vi "Get board layout.vi"(11 "Board in":refnum<class "Board.lvclass">) -> (2 "Board layout":cluster{"Occupied":bool, "Piece":T1}[][](array[cluster]), 3 "Board out":refnum<class "Board.lvclass">)   [LabVIEW 2015, in "Chesslib.lvlib" / "Board.lvclass"]
uses:
  Board.lvclass
  typedef/Piece.ctl
  typedef/Color.ctl
  typedef/Piece type.ctl
  Pieces/Piece/Piece.lvclass/Piece.ctl
  Pieces/Piece/Piece.lvclass
  Chesslib.lvlib
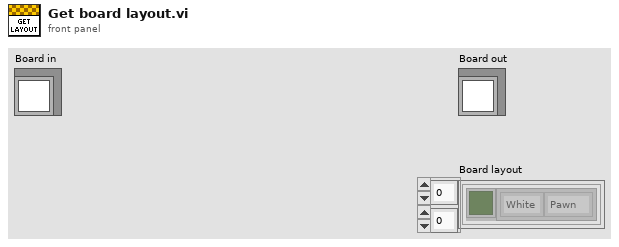
[diagram p1: front panel]
types:
  T1 = typedef "Chesslib.lvlib/Piece.ctl" = cluster{"Color":T2, "Type":T3}
  T2 = typedef "Chesslib.lvlib/Color.ctl" = enum16{"White", "Black"}
  T3 = typedef "Chesslib.lvlib/Piece type.ctl" = enum16{"Pawn", "Bishop", "Knight", "Rook", "Queen", "King"}
  T4 = cluster{"Square occupied?":bool, cluster{"Color":T2, "Piece type":T3}}
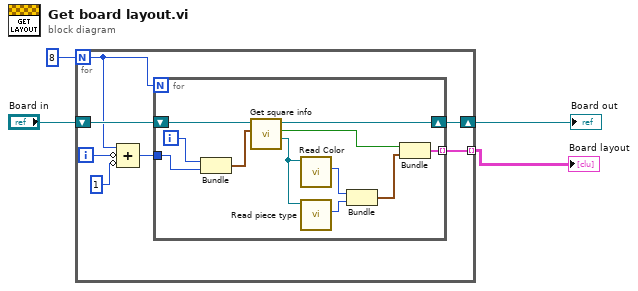
[diagram p0: block diagram]
diagram:
  n1 = for {
    N: 8 -> [w7]
    shift-right: [w10] -> w2
    shift-left: "Board in" -> [w11]
    tunnel: [w9] -> w1 mode=indexing
    i -> [w8]
    n2 = Compound Arithmetic op=ADD(w7, invert w8, invert 1 ("value")) -> (w6:i32)
    n3 = for {
      N: w7 -> [_]
      shift-right: [w21] -> w10
      shift-left: w11 -> [w22]
      tunnel: w6 -> [w13]
      tunnel: [w14] -> w9 mode=indexing
      i -> [w12]
      n4 = Bundle(w12, w13) -> (w20:cluster{i32, i32})  [unwired: 1 in]
      n5 = call "Get square info.vi"("Square"=w20, "Board in"=w22) -> ("Piece"=w18:refnum<class "Piece.lvclass">, "Square occupied?"=w19:bool, "Board out"=w21:refnum<class "Board.lvclass">)  [unwired: 7 in]
      n6 = call "Read Color.vi"("Piece in"=w18) -> ("Color"=w16:T2)  [unwired: 10 in]
      n7 = call-dynamic "Read piece type.vi"("Piece in"=w18) -> ("Piece type"=w17:T3)  [unwired: 10 in]
      n8 = Bundle("Color"=w16, "Piece type"=w17) -> (w15:cluster{"Color":T2, "Piece type":T3})  [unwired: 1 in]
      n9 = Bundle("Square occupied?"=w19, w15) -> (w14:T4)  [unwired: 1 in]
    }
  }
  "Board out" <- w2
  "Board layout" <- w1
